vi "Template - DC Power Output DC Volts.vi"() -> ()   [LabVIEW 2011]
doc: "This example shows how to configure the instrument's output voltage level, over current protection, and over voltage protection. The actual voltage level and actual current level are returned as well as whether over voltage protection (OVP) or over current protection (OCP) has been tripped."
uses:
  <instrlib>/_Template - DC Power/Template - DC Power.lvlib
panel:
  in  "Enable OVP (T: Enable)":bool=TRUE
  in  "Serial Configuration":T1={"Baud Rate"=9600, "Parity"=0, "Data Bits"=7, "Stop Bits"=10, "Flow Control"=0} {"Flow Control" items=["None", "XON/XOFF", "RTS/CTS", "XON/XOFF & RTS/CTS", "DTR/DSR", "XON/XOFF & DTR/DSR"]; "Stop Bits" items=["1.0"=10, "1.5"=15, "2.0"=20]; "Data Bits" items=["7"=7, "8"=8]; "Parity" items=["None", "Odd", "Even", "Mark", "Space"]; "Baud Rate" items=["300"=300, "600"=600, "1200"=1200, "2400"=2400, "4800"=4800, "9600"=9600, "19200"=19200]}
  in  "Stop Output":bool
  in  "Behavior (0: Regulate)":u16(ring) items=["Regulate", "Trip"]
  out "OCP Tripped?":bool
  out "OVP Tripped?":bool
  in  "Voltage Limit (0V)":dbl format="%.2f"
  out "Actual Current Limit (A)":dbl format="%.2f"
  out "Actual Voltage Level (V)":dbl format="%.2f"
  in  "Voltage Level (0.0 V)":dbl format="%.2f"
  in  "Current Limit (0A)":dbl format="%.2f"
  in  "Channel (1:Channel 1)":i32(ring)=1 items=["Channel 1"=1, "Channel 2"=2]
  in  "VISA resource name":refnum<visa-resource-name>
  # "(c) 2007 <Enter Company Name Here>.  ALL RIGHTS RESERVED."
  # "Over Voltage Protection"
  # "Over Current Protection"
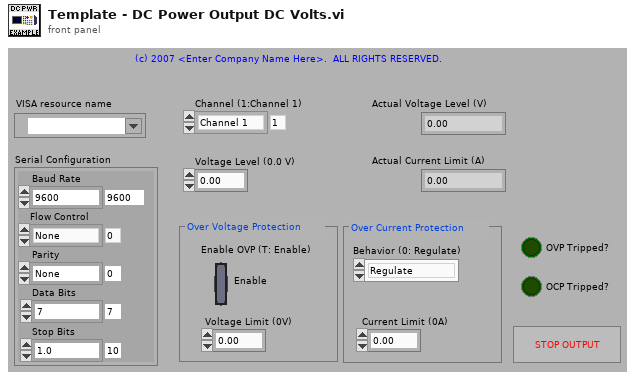
[diagram p1: front panel]
types:
  T1 = cluster{"Baud Rate":u32, "Parity":u16, "Data Bits":u16, "Stop Bits":u16, "Flow Control":u16}
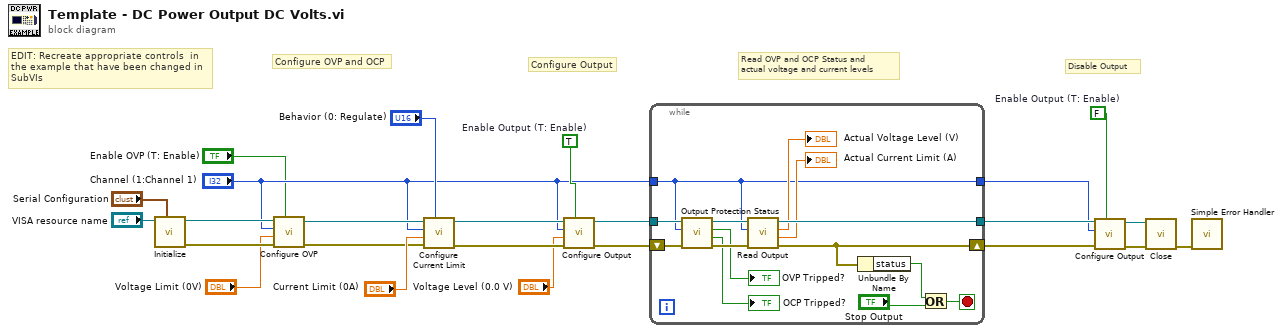
[diagram p0: block diagram]
diagram:
  w12 = FALSE  # Enable Output (T: Enable)
  w13 = TRUE  # Enable Output (T: Enable)
  # "EDIT: Recreate appropriate controls  in the example that have been changed in SubVIs"
  # "Disable Output"
  # "Read OVP and OCP Status and\nactual voltage and current levels"
  # "Configure Output"
  # "Configure OVP and OCP"
  n1 = call <instrlib>:"Initialize.vi"("Serial Configuration"="Serial Configuration", "VISA resource name"="VISA resource name") -> ("error out"=w9:errorcluster, "VISA resource name out"=w10:refnum<visa-resource-name>)  [unwired: 8 in]
  n2 = call <instrlib>:"Configure OVP.vi"("Enable OVP (T: Enable)"="Enable OVP (T: Enable)", "error in (no error)"=w9, "Voltage Limit (0.0 V)"="Voltage Limit (0V)", "Channel (1: Channel 1)"="Channel (1:Channel 1)", "VISA resource name"=w10) -> ("error out"=w8:errorcluster, "VISA resource name out"=w7:refnum<visa-resource-name>)  [unwired: 5 in]
  n3 = call <instrlib>:"Configure Current Limit.vi"("Behavior (0: Regulate)"="Behavior (0: Regulate)", "error in (no error)"=w8, "Current Limit (0.0 A)"="Current Limit (0A)", "Channel (1: Channel 1)"="Channel (1:Channel 1)", "VISA resource name"=w7) -> ("error out"=w22:errorcluster, "VISA resource name out"=w23:refnum<visa-resource-name>)  [unwired: 5 in]
  n4 = call <instrlib>:"Configure Output.vi"("Enable Output (T: Enable)"=w13, "error in (no error)"=w22, "Voltage Level (0.0 V)"="Voltage Level (0.0 V)", "Channel (1: Channel 1)"="Channel (1:Channel 1)", "VISA resource name"=w23) -> ("error out"=w19:errorcluster, "VISA resource name out"=w20:refnum<visa-resource-name>)  [unwired: 5 in]
  n5 = while {
    tunnel: w20 -> [w38]
    tunnel: [w36] -> w18
    tunnel: "Channel (1:Channel 1)" -> [w29]
    tunnel: [w29] -> w3
    shift-right: [w26] -> w17
    shift-left: w19 -> [w37]
    stop <- w28 stop-if-true
    n6 = call <instrlib>:"Output Protection Status.vi"("error in (no error)"=w37, "Channel (1: Channel 1)"=w29, "VISA resource name"=w38) -> ("error out"=w34:errorcluster, "OCP Tripped?"=→"OCP Tripped?":bool, "OVP Tripped?"=→"OVP Tripped?":bool, "VISA resource name out"=w35:refnum<visa-resource-name>)  [unwired: 5 in]
    n7 = call <instrlib>:"Read Output.vi"("error in (no error)"=w34, "Channel (1: Channel 1)"=w29, "VISA resource name"=w35) -> ("error out"=w26:errorcluster, "Actual Current Level (A)"=→"Actual Current Limit (A)":dbl, "Actual Voltage Level (V)"=→"Actual Voltage Level (V)":dbl, "VISA resource name out"=w36:refnum<visa-resource-name>)  [unwired: 5 in]
    n8 = Unbundle By Name(w26) -> ("status"=w25:bool)
    n9 = Or(x=w25, y="Stop Output") -> (x .or. y?=w28:bool)
  }
  n10 = call <instrlib>:"Configure Output.vi"("Enable Output (T: Enable)"=w12, "error in (no error)"=w17, "Channel (1: Channel 1)"=w3, "VISA resource name"=w18) -> ("error out"=w15:errorcluster, "VISA resource name out"=w16:refnum<visa-resource-name>)  [unwired: 6 in]
  n11 = call <instrlib>:"Close.vi"("error in (no error)"=w15, "VISA resource name"=w16) -> ("error out"=w11:errorcluster)  [unwired: 9 in]
  n12 = call <vilib>:"Simple Error Handler.vi"("error in (no error)"=w11) -> ()  [unwired: 4 in, 5 out]
